vi "Vision Toolkit Supported Files.vi"() -> (6 "Pattern String":string, 7 "File Extensions":string[](array[string]))   [LabVIEW 2021, in "Image.lvlib"]
doc: "Returns a string of supported image file name patterns that can be used in a File Dialog (*.tif; *.bmp; etc. and their uppercase variants) and an array of the same extensions (without the \"*\" or \".\" characters)"
uses:
  Image.lvlib
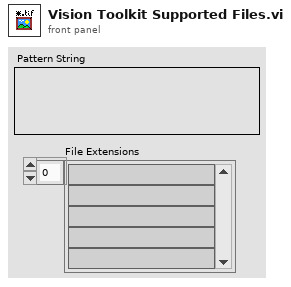
[diagram p1: front panel]
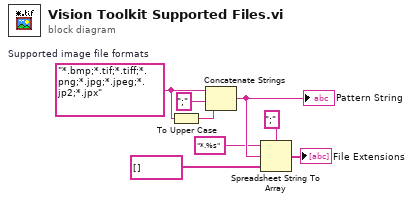
[diagram p0: block diagram]
diagram:
  w7 = "*.bmp;*.tif;*.tiff;*.png;*.jpg;*.jpeg;*.jp2;*.jpx"  # Supported image file formats
  n1 = To Upper Case(1:w7) -> (0:w8:string)
  n2 = Concatenate Strings(w7, ";" ("string"), w8) -> (w5:string)
  "Pattern String" <- w5
  n3 = Spreadsheet String To Array(delimiter (Tab)=";", format string="*.%s", spreadsheet string=w5, array type (2D Dbl)=string[] []) -> (array=→"File Extensions":string[])
